vi "myRIO v1.0 Read AI.vi"(7 "Scale Constants Array":T1, 8 "error in (no error)":errorcluster, 10 "Channel List":T5, 11 "myRIO Ref In":T3) -> (0 "error out":errorcluster, 2 "dbl Scaled Value List":dbl[](array[numeric]), 3 "myRIO Ref Out":T3)   [LabVIEW 2021]
uses:
  <vilib>/myRIO/Common/Instrument Driver Framework/myRIO v1.0/AI/typedefs/AI Channels List.ctl
  <vilib>/myRIO/Common/Instrument Driver Framework/myRIO v1.0/AI/typedefs/AI Channels Enum.ctl
  <vilib>/myRIO/Common/Instrument Driver Framework/Utilities/typedefs/myRIO v1.0 Reference.ctl
  <vilib>/myRIO/Common/Instrument Driver Framework/Utilities/typedefs/Generic FPGA Reference.ctl
  <vilib>/myRIO/Common/Instrument Driver Framework/Utilities/typedefs/Analog Scaling Constants List.ctl
  <vilib>/myRIO/Common/Instrument Driver Framework/Utilities/typedefs/Analog Scaling Constants.ctl
  <vilib>/myRIO/Common/Instrument Driver Framework/myRIO v1.0/AI/typedefs/AI Channels FPGA Reference.ctl
  <vilib>/rvi/errors/niLvFpgaAdjustHostInterfaceError.vi
  <vilib>/rvi/interface/nirviReadWriteControl/nirviReadWriteControl.xnode
  <vilib>/rvi/interface/Simulation/niFpgaSimulationCallBeginRW.vi
  NiFpgaLv.dll
panel:
  # "This VI reads one analog value from a user specified analog channel on\nthe myRIO v1.0 hardware. The value is read on the FPGA as a u16 and \nscaled to a dbl based on the specifications of the ADC. Please see Block Diagram for details."
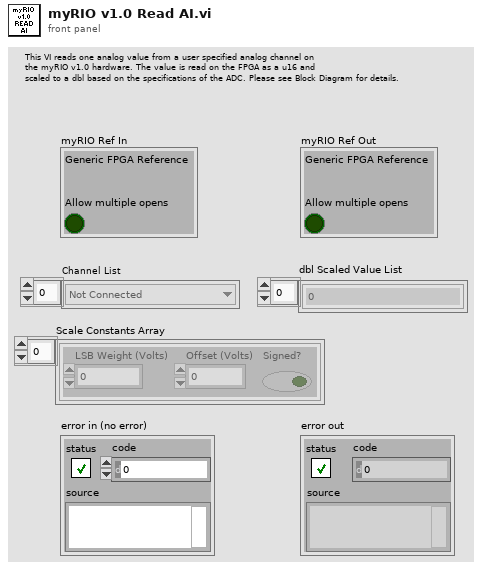
[diagram p1: front panel]
types:
  T1 = typedef "Analog Scaling Constants List.ctl" = T2[]
  T2 = typedef "Analog Scaling Constants.ctl" = cluster{"LSB Weight (Volts)":dbl, "Offset (Volts)":dbl, "Signed?":bool}
  T3 = typedef "myRIO v1.0 Reference.ctl" = cluster{"Generic FPGA Reference":T4, "Allow multiple opens":bool}
  T4 = typedef "Generic FPGA Reference.ctl" = refnum<k20>
  T5 = typedef "AI Channels List.ctl" = T6[]
  T6 = typedef "AI Channels Enum.ctl" = enum16{"Not Connected", "AudioIn/Left", "AudioIn/Right", "C/AI0", "C/AI1", "A/AI0", "A/AI1", "A/AI2", "A/AI3", "A/AI4", "A/AI5", "A/AI6", "A/AI7", "B/AI0", "B/AI1", "B/AI2", "B/AI3", "B/AI4", "B/AI5", "B/AI6", "B/AI7", "AI/AI0", "AI/AI1", "AI/AI2", "AI/AI3", "A/AI0 (DIFF)", "A/AI1 (DIFF)", "A/AI2 (DIFF)", "A/AI3 (DIFF)", "B/AI0 (DIFF)", "B/AI1 (DIFF)", "B/AI2 (DIFF)", "B/AI3 (DIFF)"}
  T7 = typedef "AI Channels FPGA Reference.ctl" = refnum<k20>
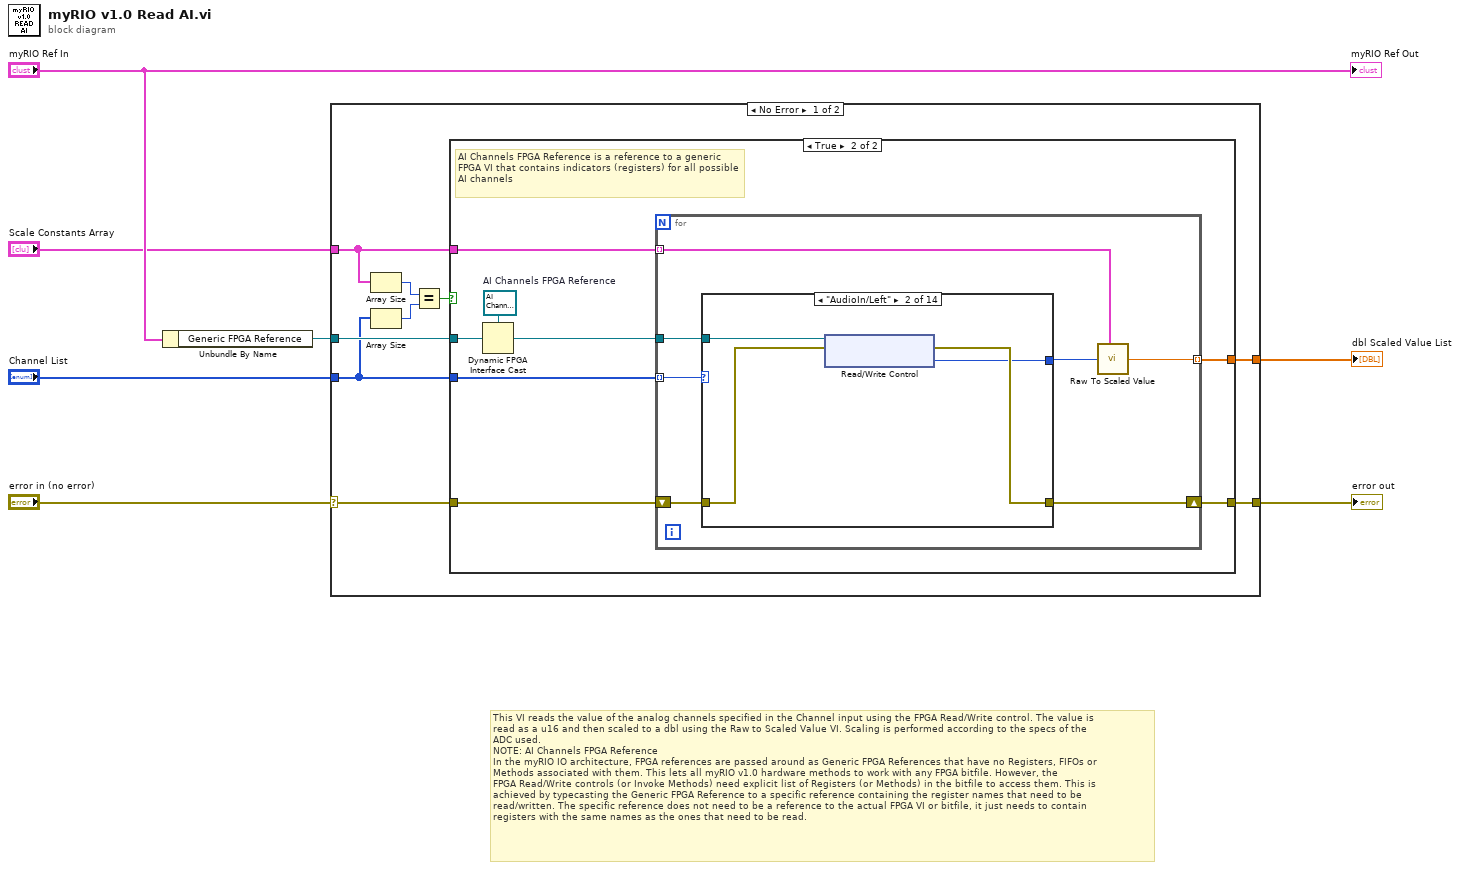
[diagram p0: block diagram]
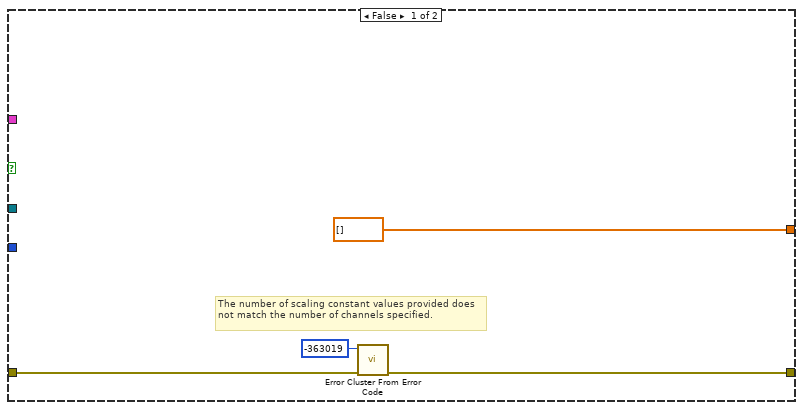
[diagram p2: hidden frame]
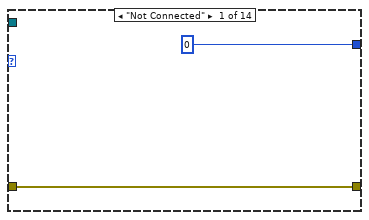
[diagram p3: hidden frame]
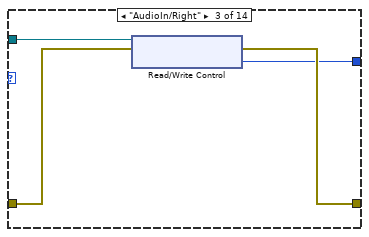
[diagram p4: hidden frame]
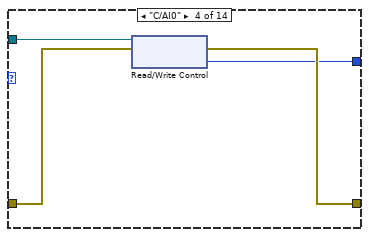
[diagram p5: hidden frame]
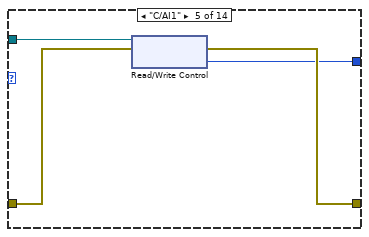
[diagram p6: hidden frame]
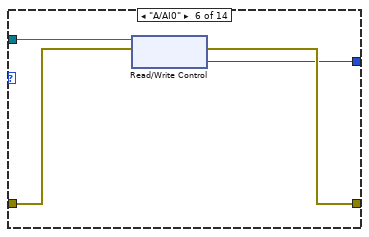
[diagram p7: hidden frame]
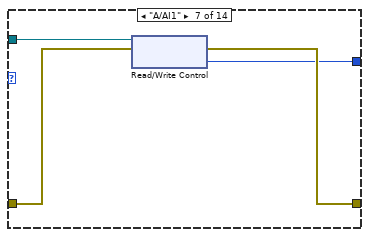
[diagram p8: hidden frame]
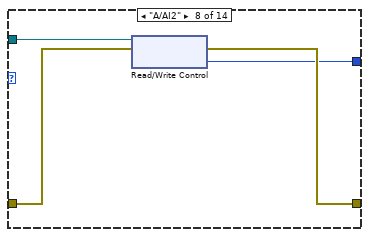
[diagram p9: hidden frame]
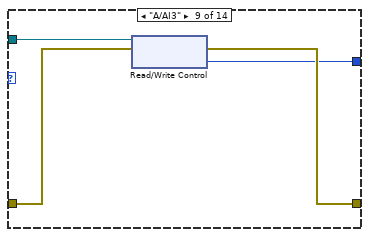
[diagram p10: hidden frame]
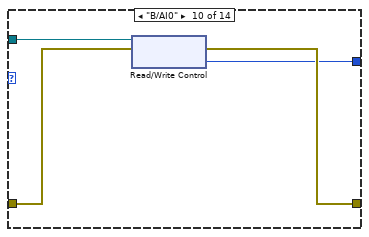
[diagram p11: hidden frame]
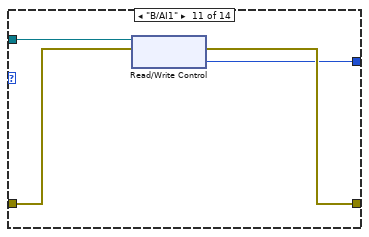
[diagram p12: hidden frame]
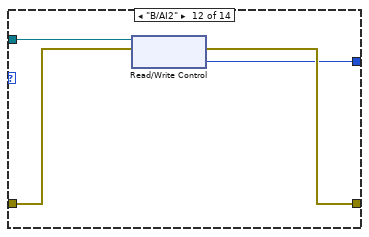
[diagram p13: hidden frame]
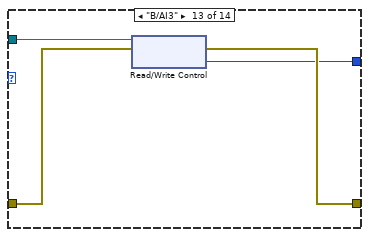
[diagram p14: hidden frame]
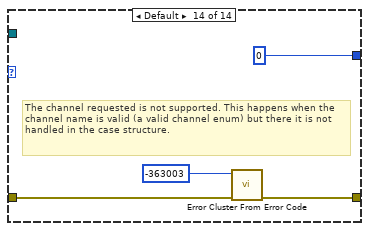
[diagram p15: hidden frame]
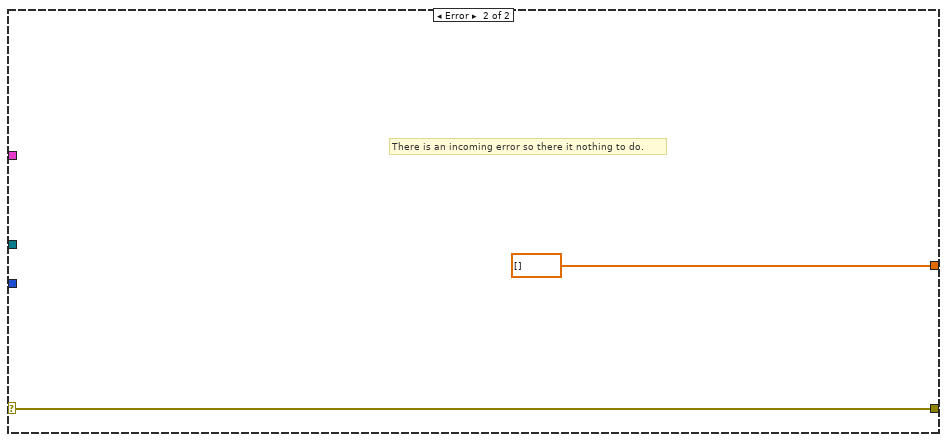
[diagram p16: hidden frame]
diagram:
  # "This VI reads the value of the analog channels specified in the Channel input using the FPGA Read/Write control. The value is \nread as a u16 and then scaled to a dbl using the Raw to Scaled Value VI. Scaling is performed according to the specs of the \nADC used.\nNOTE: AI Channels FPGA Reference\nIn the myRIO IO architecture, FPGA references are passed around as Generic FPGA References that have no Registers, FIFOs or\nMethods associated with them. This lets all myRIO v1.0 hardware methods to work with any FPGA bitfile. However, the \nFPGA Read/Write controls (or Invoke Methods) need explicit list of Registers (or Methods) in the bitfile to access them. This is \nachieved by typecasting the Generic FPGA Reference to a specific reference containing the register names that need to be \nread/written. The specific reference does not need to be a reference to the actual FPGA VI or bitfile, it just needs to contain \nregisters with the same names as the ones that need to be read."
  n1 = Unbundle By Name("myRIO Ref In") -> ("Generic FPGA Reference"=w2:T4)
  n2 = case shown="No Error" "error in (no error)" {
    selector: "error in (no error)" -> [w14 w91]
    tunnel: w2 -> [w16 _]
    tunnel: [w15 w91] -> w7
    tunnel: [w13 dbl[] []] -> w6
    tunnel: "Channel List" -> [w11 _]
    tunnel: "Scale Constants Array" -> [w12 _]
    frame No Error {
      n3 = Array Size(array=w12) -> (size(s)=w10:i32)
      n4 = Array Size(array=w11) -> (size(s)=w9:i32)
      n5 = Equal?(x=w10, y=w9) -> (x = y?=w8:bool)
      n6 = case shown="True" w8 {
        tunnel: w16 -> [_ w26]
        tunnel: [w19 w25] -> w15
        tunnel: w11 -> [_ w24]
        tunnel: w14 -> [w20 w23]
        tunnel: [dbl[] [] w22] -> w13
        tunnel: w12 -> [_ w21]
        frame False {
          # "The number of scaling constant values provided does not match the number of channels specified."
          n7 = call <vilib>:"Error Cluster From Error Code.vi"("error in (no error)"=w20, "error code (0)"=-363019) -> ("error out"=w19:errorcluster)  [unwired: 7 in]
        }
        frame True {
          w28 = T7 refnum  # AI Channels FPGA Reference
          # "AI Channels FPGA Reference is a reference to a generic FPGA VI that contains indicators (registers) for all possible AI channels"
          n8 = Dynamic FPGA Interface Cast(Session In=w28, Type=w26) -> (Session Out=w27:T7)
          n9 = for {
            tunnel: w27 -> [w35]
            shift-right: [w33] -> w25
            shift-left: w23 -> [w34]
            tunnel: w24 -> [w32] mode=indexing
            tunnel: [w30] -> w22 mode=indexing
            tunnel: w21 -> [w29] mode=indexing
            n10 = case shown="\"AudioIn/Left\"" w32 {
              tunnel: w34 -> [w37 w40 w44 w48 w52 w56 w60 w64 w68 w72 w76 w80 w84 w86]
              tunnel: [w37 w39 w43 w47 w51 w55 w59 w63 w67 w71 w75 w79 w83 w87] -> w33
              tunnel: [u16 0 ("AI7") w38 w42 w46 w50 w54 w58 w62 w66 w70 w74 w78 w82 u16 0 ("AI7")] -> w31
              tunnel: w35 -> [_ w41 w45 w49 w53 w57 w61 w65 w69 w73 w77 w81 w85 _]
              frame "Not Connected" {
              }
              frame "AudioIn/Left" {
                n11 = xnode "Read/Write Control"("FPGA VI Reference In"=w41, "error in"=w40) -> ("error out"=w39:errorcluster, "AI.AudioIn_L.VAL"=w38:u16)  [unwired: 1 out]
              }
              frame "AudioIn/Right" {
                n12 = xnode "Read/Write Control"("FPGA VI Reference In"=w45, "error in"=w44) -> ("error out"=w43:errorcluster, "AI.AudioIn_R.VAL"=w42:u16)  [unwired: 1 out]
              }
              frame "C/AI0" {
                n13 = xnode "Read/Write Control"("FPGA VI Reference In"=w49, "error in"=w48) -> ("error out"=w47:errorcluster, "AI.C_0.VAL"=w46:u16)  [unwired: 1 out]
              }
              frame "C/AI1" {
                n14 = xnode "Read/Write Control"("FPGA VI Reference In"=w53, "error in"=w52) -> ("error out"=w51:errorcluster, "AI.C_1.VAL"=w50:u16)  [unwired: 1 out]
              }
              frame "A/AI0" {
                n15 = xnode "Read/Write Control"("FPGA VI Reference In"=w57, "error in"=w56) -> ("error out"=w55:errorcluster, "AI.A_0.VAL"=w54:u16)  [unwired: 1 out]
              }
              frame "A/AI1" {
                n16 = xnode "Read/Write Control"("FPGA VI Reference In"=w61, "error in"=w60) -> ("error out"=w59:errorcluster, "AI.A_1.VAL"=w58:u16)  [unwired: 1 out]
              }
              frame "A/AI2" {
                n17 = xnode "Read/Write Control"("FPGA VI Reference In"=w65, "error in"=w64) -> ("error out"=w63:errorcluster, "AI.A_2.VAL"=w62:u16)  [unwired: 1 out]
              }
              frame "A/AI3" {
                n18 = xnode "Read/Write Control"("FPGA VI Reference In"=w69, "error in"=w68) -> ("error out"=w67:errorcluster, "AI.A_3.VAL"=w66:u16)  [unwired: 1 out]
              }
              frame "B/AI0" {
                n19 = xnode "Read/Write Control"("FPGA VI Reference In"=w73, "error in"=w72) -> ("error out"=w71:errorcluster, "AI.B_0.VAL"=w70:u16)  [unwired: 1 out]
              }
              frame "B/AI1" {
                n20 = xnode "Read/Write Control"("FPGA VI Reference In"=w77, "error in"=w76) -> ("error out"=w75:errorcluster, "AI.B_1.VAL"=w74:u16)  [unwired: 1 out]
              }
              frame "B/AI2" {
                n21 = xnode "Read/Write Control"("FPGA VI Reference In"=w81, "error in"=w80) -> ("error out"=w79:errorcluster, "AI.B_2.VAL"=w78:u16)  [unwired: 1 out]
              }
              frame "B/AI3" {
                n22 = xnode "Read/Write Control"("FPGA VI Reference In"=w85, "error in"=w84) -> ("error out"=w83:errorcluster, "AI.B_3.VAL"=w82:u16)  [unwired: 1 out]
              }
              frame Default {
                # "The channel requested is not supported. This happens when the channel name is valid (a valid channel enum) but there it is not handled in the case structure."
                n23 = call <vilib>:"Error Cluster From Error Code.vi"("error in (no error)"=w86, "error code (0)"=-363003) -> ("error out"=w87:errorcluster)  [unwired: 7 in]
              }
            }
            n24 = call <vilib>:"Raw To Scaled Value.vi"("Scaling Constants"=w29, "u16 Raw Value"=w31) -> ("dbl Scaled Value"=w30:dbl)  [unwired: 7 in]
          }
        }
      }
    }
    frame Error {
      # "There is an incoming error so there it nothing to do."
    }
  }
  "error out" <- w7
  "dbl Scaled Value List" <- w6
  "myRIO Ref Out" <- "myRIO Ref In"
